vi "calc_movement_time.vi"(4 "waiting time end (0)":u32, 5 "additional waiting time (0)":u32, 6 "Echo Mode":i32, 7 "Motor":u16(ring) items=["none", "1", "2", "3", "4", "all"], 8 "error in (no error)":errorcluster, 10 "steps":i32, 11 "VISA ressource in":refnum<visa-resource-name>="COM7") -> (0 "error out":errorcluster={"status"=FALSE, "code"=1073676294, "source"="VISA Read in write_read.vi"}, 1 "tick count":u32, 2 "move time (ms)":u32, 3 "VISA ressource out":refnum<visa-resource-name>)   [LabVIEW 2018]
uses:
  MCode_LV_86/Set Parameter.ctl
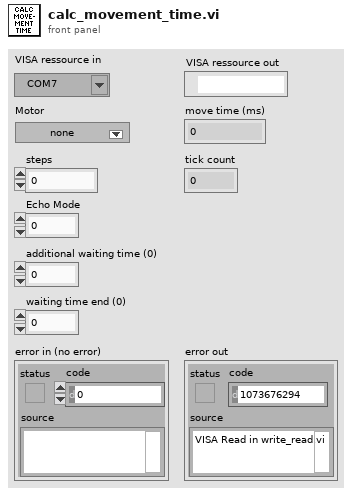
[diagram p1: front panel]
types:
  T1 = typedef "Set Parameter.ctl" = enum16{"Acceleration (A)", "Baud Rate (BD)", "Counter 1 (C1)", "Counter 2 (C2)", "Control C Software Reset (CE)", "Check Sum Enable (CK)", "Clock Mode (CM)", "Clock Mode Ratio (CR)", "Clock Mode Out Step Width (CW)", "Deceleration (D)", "Digital Filtering, Input 1 (D1)", "Digital Filtering, Input 2 (D2)", "Digital Filtering, Input 3 (D3)", "Digital Filtering, Input 4 (D4)", "Digital Filtering, Input 5 (D5)", "Digital Filtering, Input 9 (D9)", "Digital Filtering, Input 10 (D10)", "Digital Filtering, Input 11 (D11)", "Digital Filtering, Input 12 (D12)", "Deadband (DB)", "Decrement Variable (DC)", "Enable/Disable Drive (DE)", "Device Name (DN)", "End Program Execution (E)", "Encoder Function Enable (EE)", "Error Flag (EF)", "Encoder Lines (EL)", "Echo Mode (EM)", "Error Value (ER)", "Escape (ES)", "Execute Program at Address (EX)", "Firmware Version (VR)", "Hold (H)", "Hold Current (HC)", "Hold Current Delay Time (HI)", "Home to Encoder Index (HM)", "Home to Home Switch (HT)", "Increment Variable (IC)", "Initialize Parameters to NVM (IP)", "Input into Variable (IV)", "Jog Enable (JE)", "Limit Stop Mode (LM)", "Move Absolute (MA)", "Move Relative (MR)", "MicroStepping Select (MS)", "Motor Settling Delay Time (MT)", "Moving [Flag] (MV)", "Output 1 (O1)", "Output 2 (O2)", "Output 3 (O3)", "Output 4 (O4)", "Output 9 (O9)", "Output 10 (O10)", "Output 11 (O11)", "Output 12 (O12)", "Output High Byte (9-12) (OH)", "Output Low Byte (1-4) (OL)", "Output Total (1-4 and 9-12) (OT)", "Position (P)", "Position Maintenance (PM)", "Party Mode (PY)", "Register 1 (R1)", "Register 2 (R2)", "Register 3 (R3)", "Register 4 (R4)", "Reset Error(\\03)", "Run Current (RC)", "Stall Factor (SF)", "Slew (SL)", "Stall Mode Set (SM)", "Upgrade Firmware (UG)", "Velocity Initial (VI)", "Velocity Maximum (VM)", "Current1 (I1)", "Current2 (I2)", "Current3 (I3)", "Current4 (I4)", "Current5 (I5)", "Current6 (I6)", "Save (S)"}
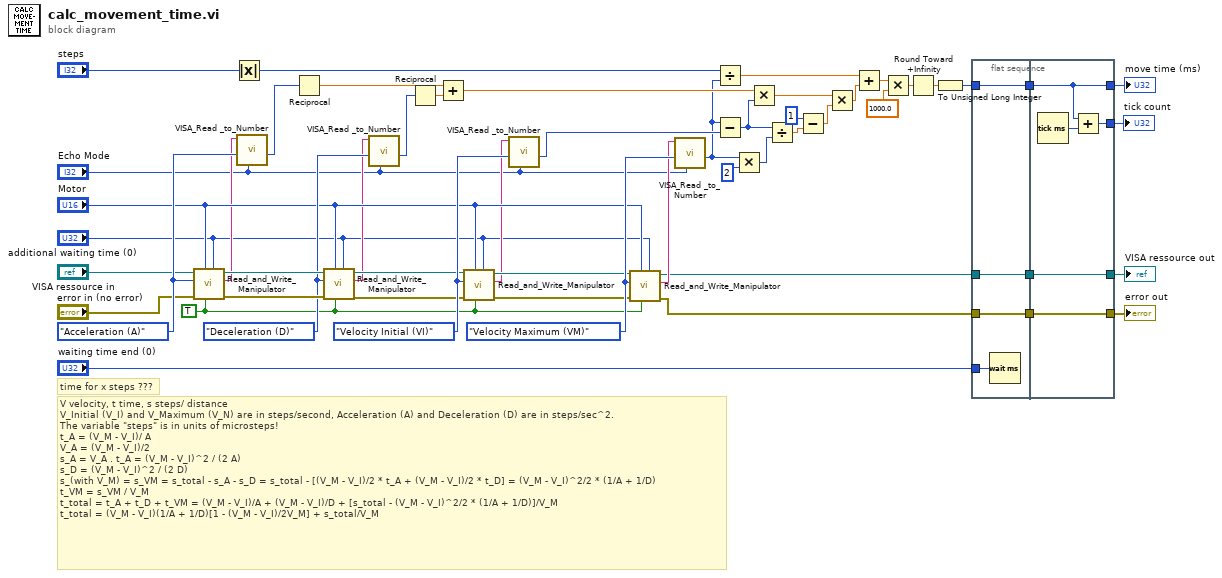
[diagram p0: block diagram]
diagram:
  w46 = Set_Parameter."Velocity Maximum (VM)" ("Command")
  w49 = Set_Parameter."Velocity Initial (VI)" ("Command")
  w24 = TRUE ("Print?")
  w50 = Set_Parameter."Deceleration (D)" ("Command")
  w51 = Set_Parameter."Acceleration (A)" ("Command")
  # "V velocity, t time, s steps/ distance\nV_Initial (V_I) and V_Maximum (V_N) are in steps/second, Acceleration (A) and Deceleration (D) are in steps/sec^2.\nThe variable \"steps\" is in units of microsteps!\nt_A = (V_M - V_I)/ A\nV_A = (V_M - V_I)/2\ns_A = V_A . t_A = (V_M - V_I)^2 / (2 A)\ns_D = (V_M - V_I)^2 / (2 D)\ns_(with V_M) = s_VM = s_total - s_A - s_D = s_total - [(V_M - V_I)/2 * t_A + (V_M - V_I)/2 * t_D] = (V_M - V_I)^2/2 * (1/A + 1/D)\nt_VM = s_VM / V_M\nt_total = t_A + t_D + t_VM = (V_M - V_I)/A + (V_M - V_I)/D + [s_total - (V_M - V_I)^2/2 * (1/A + 1/D)]/V_M\nt_total = (V_M - V_I)(1/A + 1/D)[1 - (V_M - V_I)/2V_M] + s_total/V_M"
  # "time for x steps ???"
  n1 = call "Read_and_Write_Manipulator.vi"("additional waiting time (0)"="additional waiting time (0)", "Print?"=w24, "Motor"="Motor", "error in (no error)"="error in (no error)", "Command"=w51, "VISA resource name"="VISA ressource in") -> ("error out"=w52:errorcluster, "Answer"=w23:string, "VISA ressource out"=w53:refnum<visa-resource-name>)  [unwired: 1 in, 2 out]
  n2 = Absolute Value(x="steps") -> (abs(x)=w14:i32)
  n3 = call "VISA_Read _to_Number.vi"("Echo Mode"="Echo Mode", "Command"=w51, "Answer Buffer"=w23) -> ("number (I32)"=w40:i32)  [unwired: 7 in, 1 out]
  n4 = Reciprocal(x=w40) -> (1/x=w37:dbl)
  n5 = call "Read_and_Write_Manipulator.vi"("additional waiting time (0)"="additional waiting time (0)", "Print?"=w24, "Motor"="Motor", "error in (no error)"=w52, "Command"=w50, "VISA resource name"=w53) -> ("error out"=w47:errorcluster, "Answer"=w22:string, "VISA ressource out"=w48:refnum<visa-resource-name>)  [unwired: 1 in, 2 out]
  n6 = call "VISA_Read _to_Number.vi"("Echo Mode"="Echo Mode", "Command"=w50, "Answer Buffer"=w22) -> ("number (I32)"=w39:i32)  [unwired: 7 in, 1 out]
  n7 = Reciprocal(x=w39) -> (1/x=w38:dbl)
  n8 = Add(x=w37, y=w38) -> (x+y=w36:dbl)
  n9 = call "Read_and_Write_Manipulator.vi"("additional waiting time (0)"="additional waiting time (0)", "Print?"=w24, "Motor"="Motor", "error in (no error)"=w47, "Command"=w49, "VISA resource name"=w48) -> ("error out"=w42:errorcluster, "Answer"=w21:string, "VISA ressource out"=w43:refnum<visa-resource-name>)  [unwired: 1 in, 2 out]
  n10 = call "VISA_Read _to_Number.vi"("Echo Mode"="Echo Mode", "Command"=w49, "Answer Buffer"=w21) -> ("number (I32)"=w41:i32)  [unwired: 7 in, 1 out]
  n11 = call "Read_and_Write_Manipulator.vi"("additional waiting time (0)"="additional waiting time (0)", "Print?"=w24, "Motor"="Motor", "error in (no error)"=w42, "Command"=w46, "VISA resource name"=w43) -> ("error out"=w12:errorcluster, "Answer"=w20:string, "VISA ressource out"=w9:refnum<visa-resource-name>)  [unwired: 1 in, 2 out]
  n12 = call "VISA_Read _to_Number.vi"("Echo Mode"="Echo Mode", "Command"=w46, "Answer Buffer"=w20) -> ("number (I32)"=w28:i32)  [unwired: 7 in, 1 out]
  n13 = Divide(x=w14, y=w28) -> (x/y=w35:dbl)
  n14 = Subtract(x=w28, y=w41) -> (x-y=w30:i32)
  n15 = Multiply(x=w28, y=2) -> (x*y=w27:i32)
  n16 = Multiply(x=w36, y=w30) -> (x*y=w33:dbl)
  n17 = Divide(x=w30, y=w27) -> (x/y=w26:dbl)
  n18 = Subtract(x=1, y=w26) -> (x-y=w32:dbl)
  n19 = Multiply(x=w33, y=w32) -> (x*y=w31:dbl)
  n20 = Add(x=w35, y=w31) -> (x+y=w17:dbl)
  n21 = Multiply(x=w17, y=1000.0) -> (x*y=w18:dbl)
  n22 = Round Toward +Infinity(x=w18) -> (ceil(x): smallest int >= x=w16:dbl)
  n23 = To Unsigned Long Integer(number=w16) -> (unsigned 32bit integer=w7:u32)
  n24 = flat-sequence {
    tunnel: w12 -> [w56]
    tunnel: "waiting time end (0)" -> [w57]
    tunnel: w9 -> [w55]
    tunnel: w7 -> [w54]
    tunnel: [w56] -> w4
    tunnel: [w54] -> w3
    tunnel: [w55] -> w2
    tunnel: [w61] -> w8
    tunnel: [w59] -> w6
    tunnel: [w62] -> w11
    tunnel: w4 -> [w62]
    tunnel: w3 -> [w59]
    tunnel: w2 -> [w61]
    tunnel: [w58] -> w1
    frame #0 {
      n25 = Wait (ms)(milliseconds to wait=w57) -> ()  [unwired: 1 out]
    }
    frame #1 {
      n26 = Tick Count (ms)() -> (millisecond timer value=w60:u32)
      n27 = Add(x=w59, y=w60) -> (x+y=w58:u32)
    }
  }
  "error out" <- w11
  "VISA ressource out" <- w8
  "move time (ms)" <- w6
  "tick count" <- w1
